vi "Set_reference_Point (SubVI)_v2.vi"(8 "error in (no error)":errorcluster, 11 "Application in":refnum<vi>) -> (0 "error out":errorcluster, 3 "Application out":refnum<vi>)   [LabVIEW 2014]
uses:
  <userlib>/Nanonis Prog Interface V5/Nanonis Prog Interface.lvlib
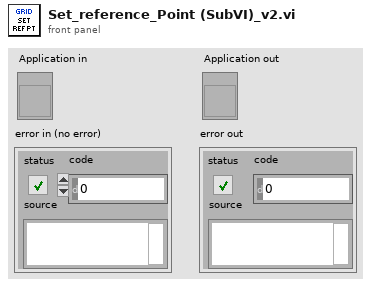
[diagram p1: front panel]
types:
  T1 = cluster{"X (m)":sgl, "Y (m)":sgl, "Text":string, "Color":u32, "Visible":bool}[]
  T2 = cluster{"x(m)":sgl, "y(m)":sgl, "Text":string, "Color":u32}
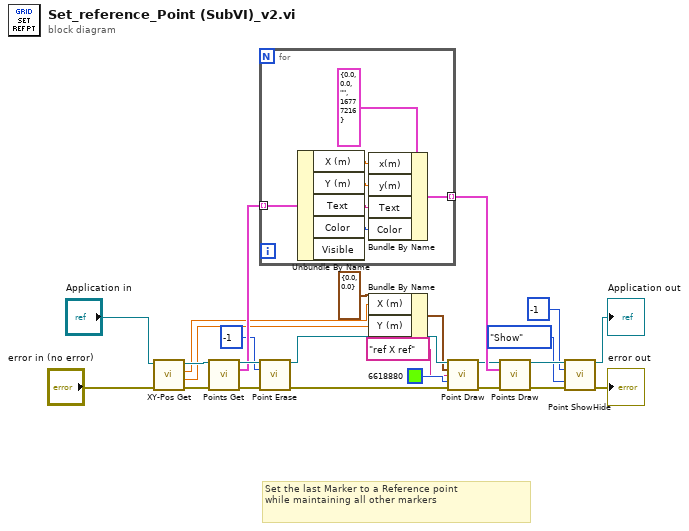
[diagram p0: block diagram]
diagram:
  # "Set the last Marker to a Reference point\nwhile maintaining all other markers"
  n1 = call <userlib>:"XY-Pos Get.vi"("error in (no error)"="error in (no error)", "Application ref in"="Application in") -> ("error out"=w6:errorcluster, "Y (m)"=w14:sgl, "X (m)"=w13:sgl, "Application ref out"=w21:refnum<vi>)  [unwired: 5 in]
  n2 = call <userlib>:"Points Get.vi"("Application ref in"=w21, "error in (no error)"=w6) -> ("Application ref out"=w22:refnum<vi>, "Points"=w20:T1, "error out"=w5:errorcluster)  [unwired: 11 in]
  n3 = for {
    tunnel: w20 -> [w32] mode=indexing
    tunnel: [w26] -> w25 mode=indexing
    n4 = Unbundle By Name(w32) -> ("X (m)"=w30:sgl, "Y (m)"=w29:sgl, "Text"=w28:string, "Color"=w27:u32)  [unwired: 1 out]
    n5 = Bundle By Name(cluster=T2 {"x(m)"=0.0, "y(m)"=0.0, "Text"="", "Color"=16777216} ("Point"), "x(m)"=w30, "y(m)"=w29, "Text"=w28, "Color"=w27) -> (w26:T2)
  }
  n6 = call <userlib>:"Point Erase.vi"("Application ref in"=w22, "Point index (-1=All points)"=-1, "error in (no error)"=w5) -> ("Application ref out"=w18:refnum<vi>, "error out"=w4:errorcluster)  [unwired: 11 in]
  n7 = Bundle By Name(cluster=cluster{"X (m)":sgl, "Y (m)":sgl} {"X (m)"=0.0, "Y (m)"=0.0} ("Point Coordinates"), "X (m)"=w13, "Y (m)"=w14) -> (w12:cluster{"X (m)":sgl, "Y (m)":sgl})
  n8 = call <userlib>:"Point Draw.vi"("Application ref in"=w18, "Point Coordinates"=w12, "Text"="ref X ref", "Color"=u32 6618880, "error in (no error)"=w4) -> ("Application ref out"=w23:refnum<vi>, "error out"=w3:errorcluster)  [unwired: 9 in]
  n9 = call <userlib>:"Points Draw.vi"("Application ref in"=w23, "Points Configuration"=w25, "error in (no error)"=w3) -> ("Application ref out"=w24:refnum<vi>, "error out"=w2:errorcluster)  [unwired: 11 in]
  n10 = call <userlib>:"Point ShowHide.vi"("Application ref in"=w24, "Point index (-1=All points)"=-1, "Show/Hide"=enum16{"Show", "Hide"}."Show", "error in (no error)"=w2) -> ("Application ref out"=→"Application out":refnum<vi>, "error out"=→"error out":errorcluster)  [unwired: 10 in]
